vi "Poll Cylinder Setpoint Control.vi"(8 "error in (no error)":errorcluster, 11 "Cylinder.lvclass":refnum<class "Cylinder.lvclass">) -> ()   [LabVIEW 2015, in "cRIO-Carbondioxide.lvlib" / "CO2-Actor.lvlib" / "Cylinder.lvclass"]
uses:
  Cylinder.lvclass
  Cylinder.lvclass/Cylinder.ctl
  <vilib>/ActorFramework/Actor/Actor.lvclass/Actor.ctl
  <vilib>/ActorFramework/Message Enqueuer/Message Enqueuer.lvclass/Message Enqueuer.ctl
  Cylinder Messages/Set Pressure Msg/Set Pressure Msg.lvclass/Set Pressure Msg.ctl
  <vilib>/ActorFramework/Actor/Read Self Enqueuer.vi
  <vilib>/ActorFramework/Message Enqueuer/Enqueue.vi
  <vilib>/ActorFramework/Message Enqueuer/Init from Existing Queue.vi
  <vilib>/ActorFramework/Message Priority Queue/Priority Enqueue.vi
  <vilib>/ActorFramework/Actor/Actor.lvclass
  <vilib>/ActorFramework/Message Enqueuer/Message Enqueuer.lvclass
  Cylinder Messages/Set Pressure Msg/Set Pressure Msg.lvclass
  CO2 Actor/CO2 Actor.lvclass
panel:
  out "error out":errorcluster
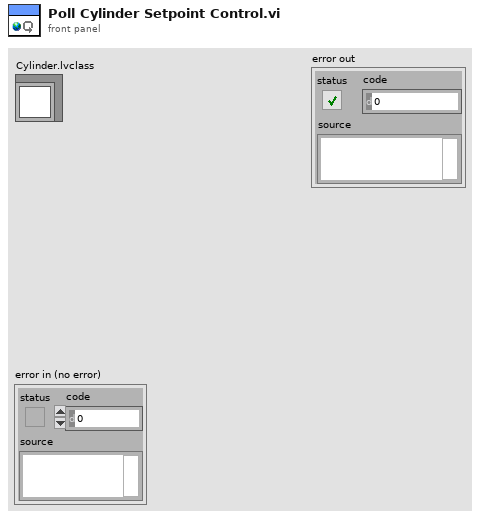
[diagram p1: front panel]
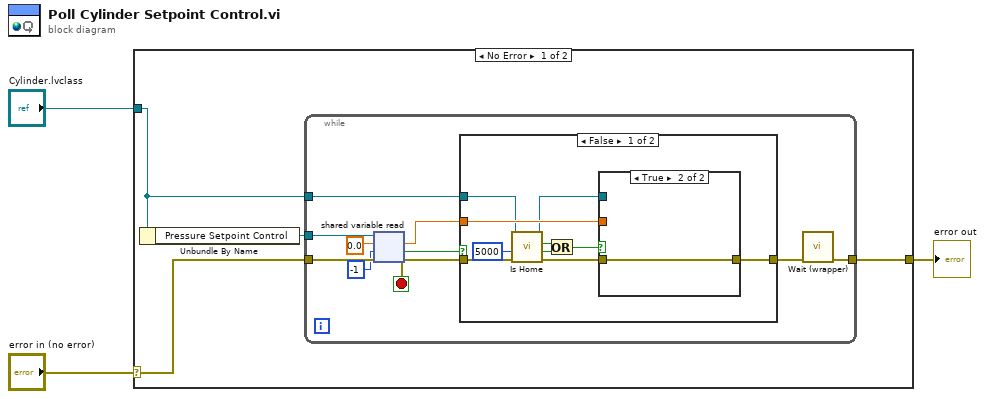
[diagram p0: block diagram]
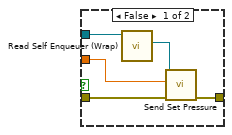
[diagram p2: hidden frame]
diagram:
  n1 = case shown="No Error" "error in (no error)" {
    selector: "error in (no error)" -> [w5 w35]
    tunnel: "Cylinder.lvclass" -> [w6 _]
    tunnel: [w4 w35] -> w1
    frame No Error {
      n2 = Unbundle By Name(w6) -> ("Pressure Setpoint Control"=w7:refnum<k21>)
      n3 = while {
        tunnel: w7 -> [w17]
        tunnel: w5 -> [w16]
        tunnel: w6 -> [w10]
        tunnel: [w8] -> w4
        stop <- w11 stop-if-true
        n4 = shared-variable-read(w17, w16, 0.0, -1 ("timeout ms")) -> (w11:errorcluster, w9:bool, w12:dbl)  [unwired: 2 out]
        n5 = case shown="False" w9 {
          tunnel: w12 -> [w24 _]
          tunnel: [w25 w34] -> w13
          tunnel: w11 -> [w27 w34]
          tunnel: w10 -> [w23 _]
          frame False {
            n6 = call "Is Home.vi"("error in (no error)"=w27, "timeout in ms (0)"=5000, "Cylinder in"=w23) -> ("error out"=w26:errorcluster, "timed out?"=w19:bool, "Cylinder is Home"=w21:bool, "Cylinder out"=w22:refnum<class "Cylinder.lvclass">)  [unwired: 5 in]
            n7 = Or(x=w21, y=w19) -> (x .or. y?=w20:bool)
            n8 = case shown="True" w20 {
              tunnel: w26 -> [w32 w33]
              tunnel: [w31 w33] -> w25
              tunnel: w24 -> [w29 _]
              tunnel: w22 -> [w28 _]
              frame False {
                n9 = call "Read Self Enqueuer (Wrap).vi"("CO2 Actor in"=w28) -> ("Actor Framework:Message Enqueuer"=w30:refnum<class "Message Enqueuer.lvclass">)  [unwired: 9 in, 1 out]
                n10 = call "Send Set Pressure.vi"("error in (no error)"=w32, "Pressure (bar)"=w29, "Message Enqueuer"=w30) -> ("error out"=w31:errorcluster)  [unwired: 7 in, 1 out]
              }
              frame True {
              }
            }
          }
          frame True {
          }
        }
        n11 = call "Wait (wrapper).vi"("error in (no error)"=w13) -> ("error out"=w8:errorcluster)  [unwired: 10 in]
      }
    }
    frame Error {
    }
  }
  "error out" <- w1
